vi "Start Lock-In Channel.vi"(7 "instance":i32, 8 "error in":errorcluster, 10 "config":cluster{"config":T1, "record length":u32}, 11 "lia host in":refnum<class "LIA Host Interface.lvclass">) -> (0 "error out":errorcluster, 3 "lia host out":refnum<class "LIA Host Interface.lvclass">)   [LabVIEW 2018, in "LIA Host Interface.lvclass"]
uses:
  LIA Host Interface.lvclass
  host/Public/lock-in settings.ctl
  host/Lock-In Amplifier Example Host.lvlib
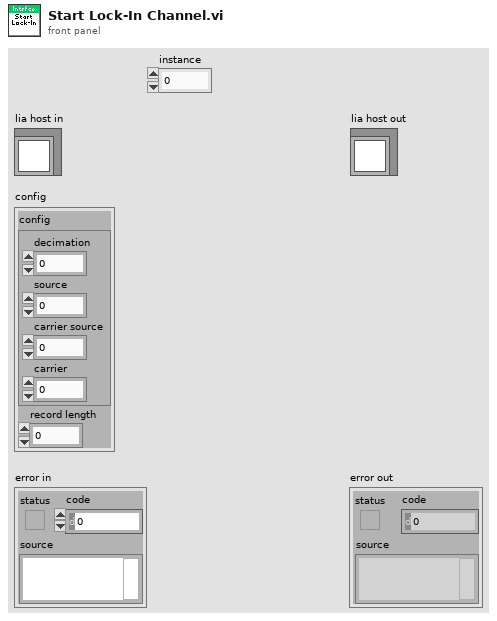
[diagram p1: front panel]
types:
  T1 = typedef "Lock-In Amplifier Example Host.lvlib/lock-in settings.ctl" = cluster{"decimation":i32, "source":i32, "carrier source":i32, "carrier":dbl}
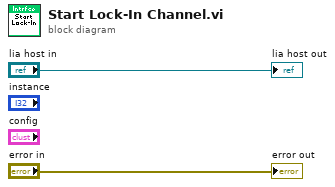
[diagram p0: block diagram]
diagram:
  "error out" <- "error in"
  "lia host out" <- "lia host in"
